vi "Write Regedit.vi"(9 "value":string caption="子项", 10 "data":string caption="新数值", 11 "subkeyName":string caption="主项") -> ()   [LabVIEW 2009]
doc: "本VI可能仅适用于Windows。\n\n本范例演示了写入Wndows注册表的方式。本VI将在本地注册表中创建一个新项并添加值。运行该VI后可以使用Read From Windows Registry.vi读取数据。从注册表读取数据后，可使用范例Delete Windows Registry Key.vi删除该项。"
uses:
  <vilib>/registry/registry.llb/Registry RtKey.ctl
  <vilib>/registry/registry.llb/Write Registry Value Simple STR.vi
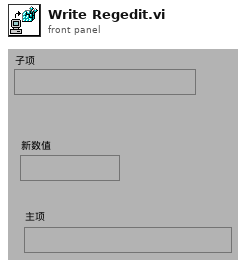
[diagram p1: front panel]
types:
  T1 = typedef "Registry RtKey.ctl" = enum32{"HKEY_CLASSES_ROOT", "HKEY_CURRENT_USER", "HKEY_LOCAL_MACHINE", "HKEY_USERS", "HKEY_PERFORMANCE_DATA", "HKEY_CURRENT_CONFIG", "HKEY_DYN_DATA"}
  T2 = typedef "Registry refnum.ctl" = refnum<k1>
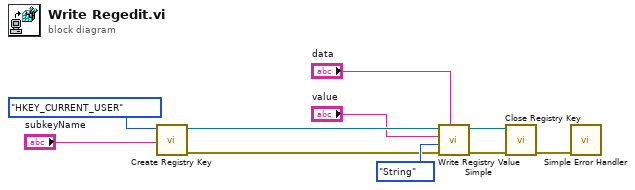
[diagram p0: block diagram]
diagram:
  n1 = call <vilib>:"Create Registry Key.vi"("subkey"="subkeyName", "root key (HKEY_LOCAL_MACHINE)"=Registry_RtKey."HKEY_CURRENT_USER") -> ("error out"=w4:errorcluster, "refnum out"=w5:T2)  [unwired: 7 in, 1 out]
  n2 = call-poly <vilib>:"Write Registry Value Simple.vi"("String/Binary data"="data", "error in (no error)"=w4, "simple data type"=enum16{"String", "Binary", "DWORD"}."String", "value"="value", "refnum"=w5) -> ("error out"=w6:errorcluster, "refnum out"=w7:T2)  [unwired: 3 in]
  n3 = call <vilib>:"Close Registry Key.vi"("error in (no error)"=w6, "refnum"=w7) -> ("error out"=w10:errorcluster)  [unwired: 5 in]
  n4 = call <vilib>:"Simple Error Handler.vi"("error in (no error)"=w10) -> ()  [unwired: 4 in, 5 out]
